vi "FTS Set Acquisition Option Single Gain.vi"(8 "error in (no error)":errorcluster, 10 "gainIndex":u16, 11 "specIndex":u16) -> (0 "error out":errorcluster, 3 "function return":i32)   [LabVIEW 2010, in "FTSLib.lvlib"]
doc: "int __cdecl FTS_SetAcquisitionOption_SingleGain(unsigned short specIndex, unsigned short gainIndex);"
uses:
  FTSLib.lvlib
  FTSLib.dll
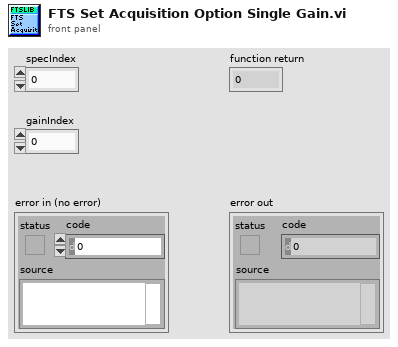
[diagram p1: front panel]
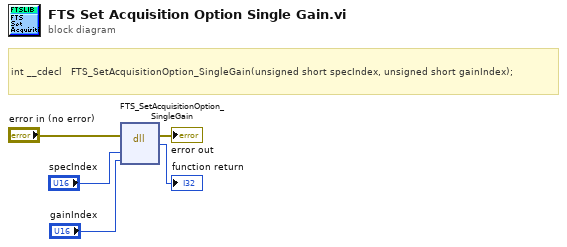
[diagram p0: block diagram]
diagram:
  # "int __cdecl   FTS_SetAcquisitionOption_SingleGain(unsigned short specIndex, unsigned short gainIndex);"
  n1 = dll-call lib="FTSLib.*" fn="FTS_SetAcquisitionOption_SingleGain"(error in="error in (no error)", "specIndex"="specIndex", "gainIndex"="gainIndex") -> (error out=→"error out":errorcluster, →"function return":i32)  [unwired: 4 in, 1 out]
